vi "experiment control.vi"() -> ()   [LabVIEW 2012] (continued)
                n2818 = Flatten To String(anything=w6200, error in (no error)=w6205) -> (data string=w6206:string, error out=w6204:errorcluster)  [unwired: 2 in, 1 out]
                n2819 = TCP Write(connection ID=w6203, data in=w6206, error in (no error)=w6204) -> (connection ID out=w6202:refnum<k5>, error out=w6207:errorcluster)  [unwired: 1 in, 1 out]
                n2820 = Enqueue Element(queue=w6209, element="Debug: Console >> Matlab is asking for documentation of commands." ("string"), error in (no error)=w6207) -> (error out=w6208:errorcluster)  [unwired: 1 in, 2 out]
              }
              frame "controls" {
                n2821 = control-ref of="This VI"() -> (w6211:refnum<vi>)
                n2822 = call "all refs.vi"("VI"=w6211) -> ("all controls"=w6212:refnum<vi>[])
                n2823 = for {
                  tunnel: w6212 -> [w6221] mode=indexing
                  tunnel: [w6220] -> w6217 mode=indexing
                  n2824 = property class="Ctl"(reference=w6221) -> ("Label.Text"=w6220:string)  [unwired: 1 in, 2 out]
                }
                n2825 = Flatten To String(anything=w6217, error in (no error)=w6214) -> (data string=w6216:string, error out=w6213:errorcluster)  [unwired: 2 in, 1 out]
                n2826 = TCP Write(connection ID=w6215, data in=w6216, error in (no error)=w6213) -> (connection ID out=w6219:refnum<k5>, error out=w6210:errorcluster)  [unwired: 1 in, 1 out]
              }
              frame "type" {
                n2827 = control-ref of="This VI"() -> (w6223:refnum<vi>)
                n2828 = TCP Read(connection ID=w6231, bytes to read=4, error in (no error)=w6230, 9:10000 ("timeout ms (25000)")) -> (connection ID out=w6235:refnum<k5>, data out=w6237:string, error out=w6236:errorcluster)  [unwired: 1 in]
                n2829 = Type Cast(type=u32 1 ("bytes to read"), x=w6237) -> (*(type *) &x=w6239:u32)
                n2830 = call "all refs.vi"("VI"=w6223) -> ("all controls"=w6222:refnum<vi>[])
                n2831 = To Long Integer(number=w6239) -> (32bit integer=w6240:i32)
                n2832 = for {
                  tunnel: w6222 -> [w6266] mode=indexing
                  tunnel: [w6265] -> w6229 mode=indexing
                  n2833 = property class="Ctl"(reference=w6266) -> ("Label.Text"=w6265:string)  [unwired: 1 in, 2 out]
                }
                n2834 = TCP Read(connection ID=w6235, bytes to read=w6240, error in (no error)=w6236) -> (connection ID out=w6228:refnum<k5>, data out=w6226:string, error out=w6227:errorcluster)  [unwired: 2 in]
                n2835 = Search 1D Array(1D array=w6229, element=w6226) -> (index of element=w6224:i32)  [unwired: 1 in]
                n2836 = Greater Or Equal To 0?(x=w6224) -> (x >= 0?=w6225:bool)
                n2837 = case shown="True" w6225 {
                  tunnel: [w6243 w6264] -> w6242
                  tunnel: [w6244 w6257] -> w6241
                  tunnel: w6232 -> [_ w6263]
                  tunnel: w6222 -> [w6256 _]
                  tunnel: w6224 -> [w6255 _]
                  tunnel: w6228 -> [w6251 w6257]
                  tunnel: w6227 -> [w6250 w6258]
                  tunnel: w6226 -> [_ w6260]
                  frame True {
                    n2838 = Index Array(array=w6256, index=w6255) -> (element=w6254:refnum<vi>)
                    n2839 = property class="Ctl"(reference=w6254) -> ("Value"=w6246:variant)  [unwired: 1 in, 2 out]
                    n2840 = call "ubinary_single.vi"("Cluster"=w6246) -> ("Header"=w6245:cluster{"Element Names":string[], u8[]})  [unwired: 9 in, 1 out]
                    n2841 = Flatten To String(anything=w6245) -> (data string=w6248:string)  [unwired: 3 in, 2 out]
                    n2842 = String Length(string=w6248) -> (length=w6247:i32)
                    n2843 = Flatten To String(anything=w6247) -> (data string=w6249:string)  [unwired: 3 in, 2 out]
                    n2844 = TCP Write(connection ID=w6251, data in=w6249, error in (no error)=w6250) -> (connection ID out=w6252:refnum<k5>, error out=w6253:errorcluster)  [unwired: 1 in, 1 out]
                    n2845 = TCP Write(connection ID=w6252, data in=w6248, error in (no error)=w6253) -> (connection ID out=w6244:refnum<k5>, error out=w6243:errorcluster)  [unwired: 1 in, 1 out]
                  }
                  frame False {
                    n2846 = Concatenate Strings("Debug: Console >> Matlab is trying to read type of control " ("string"), w6260, ", but it doesn't exist!" ("string")) -> (w6261:string)
                    n2847 = Enqueue Element(queue=w6263, element=w6261, error in (no error)=w6258) -> (error out=w6264:errorcluster)  [unwired: 1 in, 2 out]
                  }
                }
              }
              frame "read" {
                n2848 = control-ref of="This VI"() -> (w6268:refnum<vi>)
                n2849 = TCP Read(connection ID=w6276, bytes to read=4, error in (no error)=w6275, 9:10000 ("timeout ms (25000)")) -> (connection ID out=w6280:refnum<k5>, data out=w6282:string, error out=w6281:errorcluster)  [unwired: 1 in]
                n2850 = Type Cast(type=u32 1 ("bytes to read"), x=w6282) -> (*(type *) &x=w6284:u32)
                n2851 = call "all refs.vi"("VI"=w6268) -> ("all controls"=w6267:refnum<vi>[])
                n2852 = To Long Integer(number=w6284) -> (32bit integer=w6285:i32)
                n2853 = for {
                  tunnel: w6267 -> [w6310] mode=indexing
                  tunnel: [w6309] -> w6274 mode=indexing
                  n2854 = property class="Ctl"(reference=w6310) -> ("Label.Text"=w6309:string)  [unwired: 1 in, 2 out]
                }
                n2855 = TCP Read(connection ID=w6280, bytes to read=w6285, error in (no error)=w6281) -> (connection ID out=w6273:refnum<k5>, data out=w6271:string, error out=w6272:errorcluster)  [unwired: 2 in]
                n2856 = Search 1D Array(1D array=w6274, element=w6271) -> (index of element=w6269:i32)  [unwired: 1 in]
                n2857 = Greater Or Equal To 0?(x=w6269) -> (x >= 0?=w6270:bool)
                n2858 = case shown="True" w6270 {
                  tunnel: [w6288 w6308] -> w6287
                  tunnel: [w6300 w6301] -> w6286
                  tunnel: w6277 -> [_ w6307]
                  tunnel: w6267 -> [w6297 _]
                  tunnel: w6269 -> [w6296 _]
                  tunnel: w6273 -> [w6289 w6301]
                  tunnel: w6272 -> [w6290 w6302]
                  tunnel: w6271 -> [_ w6304]
                  frame True {
                    n2859 = Index Array(array=w6297, index=w6296) -> (element=w6295:refnum<vi>)
                    n2860 = property class="Ctl"(reference=w6295) -> ("Value"=w6291:variant)  [unwired: 1 in, 2 out]
                    n2861 = Variant To Flattened String(Variant=w6291) -> (data string=w6292:string)  [unwired: 1 out]
                    n2862 = String Length(string=w6292) -> (length=w6294:i32)
                    n2863 = Flatten To String(anything=w6294) -> (data string=w6293:string)  [unwired: 3 in, 2 out]
                    n2864 = TCP Write(connection ID=w6289, data in=w6293, error in (no error)=w6290) -> (connection ID out=w6299:refnum<k5>, error out=w6298:errorcluster)  [unwired: 1 in, 1 out]
                    n2865 = TCP Write(connection ID=w6299, data in=w6292, error in (no error)=w6298) -> (connection ID out=w6300:refnum<k5>, error out=w6288:errorcluster)  [unwired: 1 in, 1 out]
                  }
                  frame False {
                    n2866 = Concatenate Strings("Debug: Console >> Matlab is trying to read the control " ("string"), w6304, ", but it doesn't exist!" ("string")) -> (w6305:string)
                    n2867 = Enqueue Element(queue=w6307, element=w6305, error in (no error)=w6302) -> (error out=w6308:errorcluster)  [unwired: 1 in, 2 out]
                  }
                }
              }
              frame "write" {
                n2868 = control-ref of="This VI"() -> (w6312:refnum<vi>)
                n2869 = TCP Read(connection ID=w6320, bytes to read=4, error in (no error)=w6319, 9:10000 ("timeout ms (25000)")) -> (connection ID out=w6324:refnum<k5>, data out=w6326:string, error out=w6325:errorcluster)  [unwired: 1 in]
                n2870 = Type Cast(type=u32 1 ("bytes to read"), x=w6326) -> (*(type *) &x=w6328:u32)
                n2871 = call "all refs.vi"("VI"=w6312) -> ("all controls"=w6311:refnum<vi>[])
                n2872 = To Long Integer(number=w6328) -> (32bit integer=w6329:i32)
                n2873 = for {
                  tunnel: w6311 -> [w6363] mode=indexing
                  tunnel: [w6362] -> w6318 mode=indexing
                  n2874 = property class="Ctl"(reference=w6363) -> ("Label.Text"=w6362:string)  [unwired: 1 in, 2 out]
                }
                n2875 = TCP Read(connection ID=w6324, bytes to read=w6329, error in (no error)=w6325) -> (connection ID out=w6317:refnum<k5>, data out=w6315:string, error out=w6316:errorcluster)  [unwired: 2 in]
                n2876 = Search 1D Array(1D array=w6318, element=w6315) -> (index of element=w6313:i32)  [unwired: 1 in]
                n2877 = Greater Or Equal To 0?(x=w6313) -> (x >= 0?=w6314:bool)
                n2878 = case shown="True" w6314 {
                  tunnel: [w6332 w6361] -> w6331
                  tunnel: [w6337 w6354] -> w6330
                  tunnel: w6321 -> [_ w6360]
                  tunnel: w6311 -> [w6353 _]
                  tunnel: w6313 -> [w6352 _]
                  tunnel: w6317 -> [w6339 w6354]
                  tunnel: w6316 -> [w6340 w6355]
                  tunnel: w6315 -> [_ w6357]
                  frame True {
                    n2879 = TCP Read(connection ID=w6339, bytes to read=4, error in (no error)=w6340, 9:10000 ("timeout ms (25000)")) -> (connection ID out=w6346:refnum<k5>, data out=w6344:string, error out=w6345:errorcluster)  [unwired: 1 in]
                    n2880 = Index Array(array=w6353, index=w6352) -> (element=w6351:refnum<vi>)
                    n2881 = Type Cast(type=u32 1 ("bytes to read"), x=w6344) -> (*(type *) &x=w6342:u32)
                    n2882 = property class="Ctl"(reference=w6351) -> (reference out=w6334:refnum<vi>, error out=w6333:errorcluster, "Value"=w6350:variant)  [unwired: 1 in]
                    n2883 = To Long Integer(number=w6342) -> (32bit integer=w6341:i32)
                    n2884 = Variant To Flattened String(Variant=w6350) -> (1:w6349:i16[])  [unwired: 1 out]
                    n2885 = TCP Read(connection ID=w6346, bytes to read=w6341, error in (no error)=w6345) -> (connection ID out=w6337:refnum<k5>, data out=w6338:string, error out=w6332:errorcluster)  [unwired: 2 in]
                    n2886 = Flattened String To Variant(4:w6333, 6:w6338, 7:w6349) -> (0:w6335:errorcluster, 3:w6336:variant)
                    n2887 = property class="Ctl"(reference=w6334, error in=w6335, "Value"=w6336) -> ()  [unwired: 2 out]
                  }
                  frame False {
                    n2888 = Concatenate Strings("Debug: Console >> Matlab is trying to write to control " ("string"), w6357, ", but it doesn't exist!" ("string")) -> (w6358:string)
                    n2889 = Enqueue Element(queue=w6360, element=w6358, error in (no error)=w6355) -> (error out=w6361:errorcluster)  [unwired: 1 in, 2 out]
                  }
                }
              }
              frame "sync" {
                # "Rendezvous at the \"sync\" point. If the primary event loop is in the \"Sync\" state, then this will allow the primary event loop to continue. Returns 1 If the main loop was waiting in the Sync state, and 1   if it wasn't. This allows Matlab to wait for Sync."
                n2890 = call <vilib>:"Create Rendezvous.vi"("error in (no error)"=w6369, "return existing (F)"=TRUE, "name (unnamed)"="sync") -> ("error out"=w6367:errorcluster, "rendezvous"=w6371:T56)  [unwired: 2 in, 1 out]
                n2891 = case shown="No Error" w6367 {
                  tunnel: w6371 -> [w6379 _]
                  tunnel: w6367 -> [w6378 w6380]
                  tunnel: [w6376 w6384] -> w6368
                  tunnel: [w6374 w6383] -> w6364
                  tunnel: w6365 -> [w6373 w6382]
                  frame No Error {
                    n2892 = call <vilib>:"Wait at Rendezvous.vi"("error in (no error)"=w6378, "rendezvous"=w6379) -> ("error out"=w6375:errorcluster)  [unwired: 3 in, 2 out]
                    n2893 = TCP Write(connection ID=w6373, data in="\u0001", error in (no error)=w6375) -> (connection ID out=w6374:refnum<k5>, error out=w6376:errorcluster)  [unwired: 1 in, 1 out]
                  }
                  frame Error {
                    n2894 = call <vilib>:"Clear Errors.vi"("error in (no error)"=w6380) -> ("error out"=w6385:errorcluster)  [unwired: 6 in]
                    n2895 = TCP Write(connection ID=w6382, data in="\u0000", error in (no error)=w6385) -> (connection ID out=w6383:refnum<k5>, error out=w6384:errorcluster)  [unwired: 1 in, 1 out]
                  }
                }
              }
            }
            n2896 = TCP Close Connection(connection ID=w6165, error in (no error)=w6166) -> ()  [unwired: 1 in, 2 out]
          }
          frame Error {
          }
        }
        n2897 = Get Queue Status(queue=w6158, return elements? (F)=TRUE) -> (error out=w6164:errorcluster, elements=→"queue":string[])  [unwired: 1 in, 6 out]
      }
    }
    frame Disabled {
    }
  }
  n2898 = Release Queue(queue=w4, error in (no error)=w3) -> (error out=w2:errorcluster)  [unwired: 1 in, 2 out]
  n2899 = call <vilib>:"Clear Errors.vi"("error in (no error)"=w2) -> ()  [unwired: 6 in, 1 out]
